vi "全局-被反馈配置.vi"() -> ()   [LabVIEW 2019]
panel:
  in  "启用反馈？":bool=TRUE
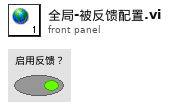
[diagram p1: front panel]
diagram:
